vi "solar_voy VoyagerIDOffset Lookup.vi"(8 "error in (no error)":errorcluster, 10 "Target Name":string, 11 "Voyager Refnum in":T1) -> (0 "error out":errorcluster, 2 "VoyagerIDOffset":u16, 3 "Voyager Refnum out":T1)   [LabVIEW 2018]
doc: "Looks up an ID offset by a target name."
uses:
  solar_voy_ctl Voyager Refnum.ctl
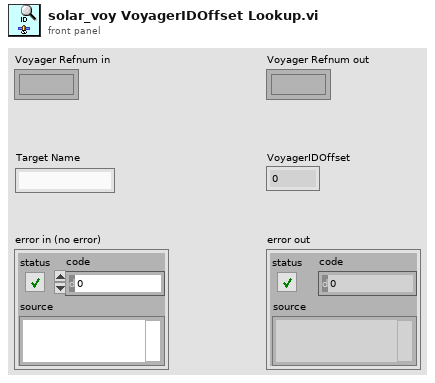
[diagram p1: front panel]
types:
  T1 = typedef "solar_voy_ctl Voyager Refnum.ctl" = refnum<k1>
  T2 = typedef "solar_voy_ctl Voyager.ctl" = cluster{"PACKETS":T3[], "COSMOS_Root":path, "CMD_HDR":T8, "TLM_HDR":T8, "TCPs":T9[], "VoyagerIDOffset":cluster{"VoyagerIDOffset":u16[], "Target Names":string[]}}
  T3 = typedef "solar_voy_def_ctl PACKET.ctl" = cluster{"PACKET_ID":T4, "ENDIAN":enum8{"BIG", "LITTLE"}, "DESC":string, "HZRD":bool, "ITEMS":T5[], "NoExport":bool, "last_time":timestamp, "last_count":u32, "last_data":string}
  T4 = typedef "solar_voy_def_ctl PACKET_ID.ctl" = cluster{"ID":u16, "CMD":enum8{"CMD", "TLM"}, "TARGET":string, "PACKET":string}
  T5 = typedef "solar_voy_def_ctl ITEM.ctl" = cluster{"NAME":string, "OFFSET":i32, "SIZE":i32, "TYPE":T6, "EACH_SIZE":i32, "LVTYPE":T7, "MIN":dbl, "MAX":dbl, "DEFAULT":string, "DESC":string, "ID":bool, "MODIFIERS":variant, "last_value":variant}
  T6 = typedef "solar_voy_def_ctl ITEM TYPE.ctl" = enum8{"BLOCK", "INT", "UINT", "FLOAT", "STRING"}
  T7 = typedef "solar_type Item Type.ctl" = enum16{"NULL", "UNKNOWN", "CLUSTER", "I8", "I16", "I32", "I64", "U8", "U16", "U32", "U64", "U8_ENUM", "U16_ENUM", "U32_ENUM", "SGL", "DBL", "BOOLEAN", "STRING", "PATH", "VISA", "TAG", "TIME", "I8_1D", "I16_1D", "I32_1D", "I64_1D", "U8_1D", "U16_1D", "U32_1D", "U64_1D", "U8_ENUM_1D", "U16_ENUM_1D", "U32_ENUM_1D", "SGL_1D", "DBL_1D", "BOOLEAN_1D", "STRING_1D", "PATH_1D", "VISA_1D", "TAG_1D", "TIME_1D", "I8_2D", "I16_2D", "I32_2D", "I64_2D", "U8_2D", "U16_2D", "U32_2D", "U64_2D", "U8_ENUM_2D", "U16_ENUM_2D", "U32_ENUM_2D", "SGL_2D", "DBL_2D", "BOOLEAN_2D", "STRING_2D", "PATH_2D", "VISA_2D", "TAG_2D", "TIME_2D"}
  T8 = typedef "solar_voy_def_ctl HDR.ctl" = cluster{"ITEMS":T5[], "LENGTH_NAME":string, "LENGTH_VALUE_OFFSET":i32, "ID_NAME":string, "ENDIAN":enum8{"BIG", "LITTLE"}, "GUID_NAME":string, "DEFAULT_TARGET":string, "DEFAULT_PACKET":string, "DEFAULT_ERROR":string}
  T9 = typedef "solar_voy_ctl TCP.ctl" = cluster{"Connected":bool, "Port":u16, "Listener":refnum<k5>, "ServerIP":string, "TCP":refnum<k5>, "Setup":T10, "VIRefnum":refnum<vi>, "TARGETS_CMD":string[], "TARGETS_TLM":string[]}
  T10 = typedef "solar_voy_ctl Port Setup.ctl" = enum8{"SERVER", "CLIENT", "SERVER_CMD", "SERVER_TLM"}
  T11 = cluster{"VoyagerIDOffset":u16[], "Target Names":string[]}
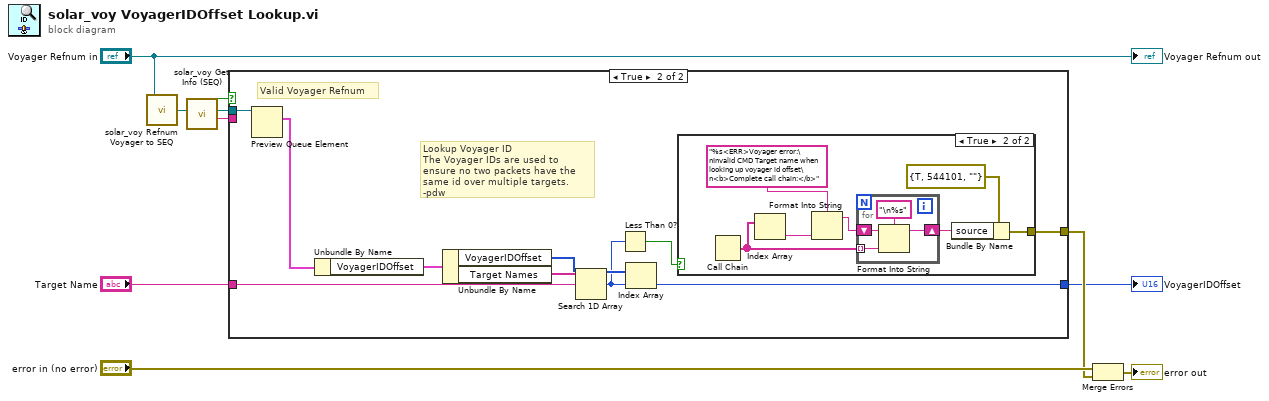
[diagram p0: block diagram]
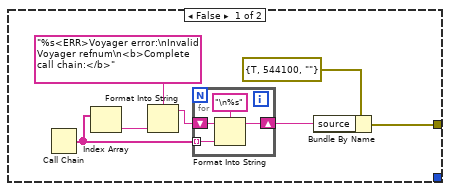
[diagram p2: hidden frame]
diagram:
  n1 = call "solar_voy Refnum Voyager to SEQ.vi"("Voyager Refnum"="Voyager Refnum in") -> ("Voyager SEQ"=w7:refnum<queue>)
  n2 = call "solar_voy Get Info (SEQ).vi"("Voyager SEQ in"=w7) -> ("Interface Name"=w9:string, "Voyager SEQ out"=w8:refnum<queue>, "Valid?"=w10:bool)  [unwired: 8 in]
  n3 = case shown="True" w10 {
    tunnel: w8 -> [_ w31]
    tunnel: w9 -> [_ _]
    tunnel: [w11 w29] -> w3
    tunnel: "Target Name" -> [_ w28]
    tunnel: [_ w22] -> w1
    frame False {
      n4 = Call Chain() -> (call chain=w14:string[])
      n5 = Index Array(array=w14) -> (element=w16:string)  [unwired: 1 in]
      n6 = Format Into String(format string="%s<ERR>Voyager error:\nInvalid Voyager refnum\n<b>Complete call chain:</b>", w16) -> (resulting string=w15:string)  [unwired: 2 in, 1 out]
      n7 = for {
        tunnel: w14 -> [w21] mode=indexing
        shift-right: [w20] -> w13
        shift-left: w15 -> [w19]
        n8 = Format Into String(format string="\n%s", initial string=w19, w21) -> (resulting string=w20:string)  [unwired: 1 in, 1 out]
      }
      n9 = Bundle By Name(cluster=errorcluster {"status"=TRUE, "code"=544100, "source"=""} ("error in (no error)"), "source"=w13) -> (w11:errorcluster)
    }
    frame True {
      # "Lookup Voyager ID\nThe Voyager IDs are used to ensure no two packets have the same id over multiple targets. -pdw"
      # "Valid Voyager Refnum"
      n10 = Preview Queue Element(queue=w31) -> (element=w30:T2)  [unwired: 2 in, 3 out]
      n11 = Unbundle By Name(w30) -> ("VoyagerIDOffset"=w23:T11)
      n12 = Unbundle By Name(w23) -> ("VoyagerIDOffset"=w26:u16[], "Target Names"=w27:string[])
      n13 = Search 1D Array(1D array=w27, element=w28) -> (index of element=w25:i32)  [unwired: 1 in]
      n14 = Less Than 0?(x=w25) -> (x < 0?=w24:bool)
      n15 = Index Array(array=w26, index=w25) -> (element=w22:u16)
      n16 = case shown="True" w24 {
        tunnel: [_ w32] -> w29
        frame False {
        }
        frame True {
          n17 = Call Chain() -> (call chain=w35:string[])
          n18 = Index Array(array=w35) -> (element=w37:string)  [unwired: 1 in]
          n19 = Format Into String(format string="%s<ERR>Voyager error:\nInvalid CMD Target name when looking up voyager id offset\n<b>Complete call chain:</b>", w37) -> (resulting string=w36:string)  [unwired: 2 in, 1 out]
          n20 = for {
            tunnel: w35 -> [w42] mode=indexing
            shift-right: [w41] -> w34
            shift-left: w36 -> [w40]
            n21 = Format Into String(format string="\n%s", initial string=w40, w42) -> (resulting string=w41:string)  [unwired: 1 in, 1 out]
          }
          n22 = Bundle By Name(cluster=errorcluster {"status"=TRUE, "code"=544101, "source"=""} ("error in (no error)"), "source"=w34) -> (w32:errorcluster)
        }
      }
    }
  }
  "VoyagerIDOffset" <- w1
  n23 = Merge Errors("error in (no error)", w3) -> (→"error out":errorcluster)
  "Voyager Refnum out" <- "Voyager Refnum in"
